vi "Get System Time.vi"() -> (5 "Time (ns)":i64)   [LabVIEW 2021, in "Time_CIF_U.lvlib"]
doc: "System time is defined as the OS time in TAI format. It is the basis for all other times/clocks and can be used to derive them. This VI is a wrapper to provide flexibility to change to other mechanisms to get OS TAI time if needed in the future."
uses:
  Time_CIF_U.lvlib
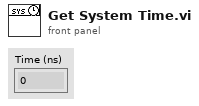
[diagram p1: front panel]
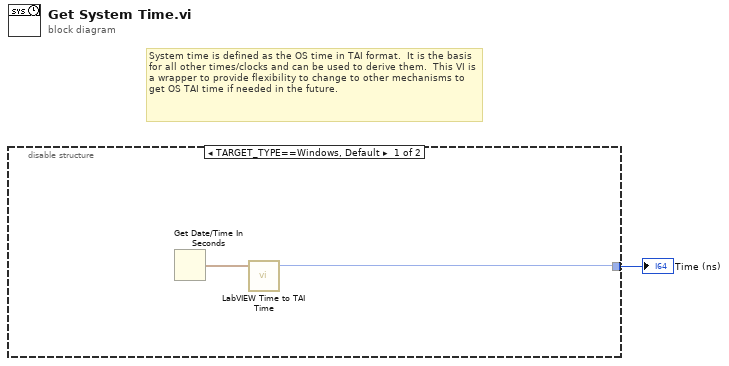
[diagram p0: block diagram]
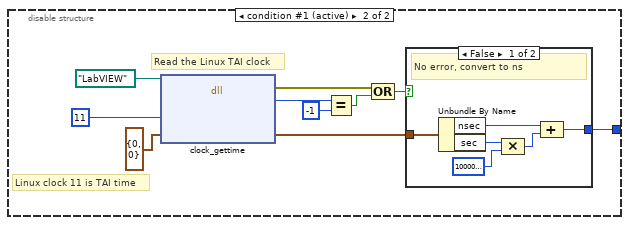
[diagram p2: hidden frame]
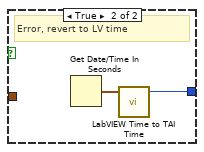
[diagram p3: hidden frame]
diagram:
  # "System time is defined as the OS time in TAI format.  It is the basis for all other times/clocks and can be used to derive them.  This VI is a wrapper to provide flexibility to change to other mechanisms to get OS TAI time if needed in the future."
  n1 = disable-structure shown="TARGET_TYPE==Windows, Default" {
    disable-tunnel: [w2 w5] -> w1
    frame condition #0 {
      n2 = Get Date/Time In Seconds() -> (seconds since 1Jan1904=w3:timestamp)
      n3 = call "LabVIEW Time to TAI Time.vi"("LabVIEW Time (s)"=w3) -> ("TAI Time (ns)"=w2:i64)  [unwired: 4 in]
    }
    frame condition #1 (active) {
      # "Read the Linux TAI clock"
      # "Linux clock 11 is TAI time"
      n4 = dll-call lib="lib/libc.so.6" fn="clock_gettime"(path in=path "LabVIEW" ("Path"), "clock_id"=u32 11, "timespec"=cluster{"sec":i64, "nsec":i64} {"sec"=0, "nsec"=0}) -> (error out=w8:errorcluster, "status"=w13:i32, "timespec"=w6:cluster{"sec":i64, "nsec":i64})  [unwired: 3 in, 1 out]
      n5 = Equal?(x=w13, y=-1) -> (x = y?=w9:bool)
      n6 = Compound Arithmetic op=OR(w8, w9) -> (w7:bool)
      n7 = case shown="False" w7 {
        tunnel: w6 -> [w17 _]
        tunnel: [w14 w20] -> w5
        frame False {
          # "No error, convert to ns"
          n8 = Unbundle By Name(w17) -> ("nsec"=w16:i64, "sec"=w19:i64)
          n9 = Compound Arithmetic op=MULTIPLY(w19, i64 1000000000 ("x")) -> (w15:i64)
          n10 = Compound Arithmetic op=ADD(w16, w15) -> (w14:i64)
        }
        frame True {
          # "Error, revert to LV time"
          n11 = Get Date/Time In Seconds() -> (seconds since 1Jan1904=w21:timestamp)
          n12 = call "LabVIEW Time to TAI Time.vi"("LabVIEW Time (s)"=w21) -> ("TAI Time (ns)"=w20:i64)  [unwired: 4 in]
        }
      }
    }
  }
  "Time (ns)" <- w1
